vi "Main.vi"(11 "Module Admin":refnum<class "Delacor_lib_QMH_Cloneable Module Admin.lvclass">) -> ()   [LabVIEW 2020, in "TCP Client.lvlib"]
doc: "This template is based off of the Queued Message Handler design pattern and the Queued Message Handler project template that ships with LabVIEW.\n\nThe main difference is that the queue is private to this module and communication between modules is performed via Broadcast and Request events.\n\nRequest events are wrapped in public API methods and are handled in the Event Handling Loop (EHL) of this VI. Any module can register for Broadcast events sent by this module. The EHL generates messages based on user interface actions.\n\nThe Message Handling Loop (MHL) processes messages generated by the EHL, or by other messages. The messages are string values, so new messages can be added easily to the Message Cases case structure in the MHL. Each message cluster can also provide an optional value for Message Data, which is a variant that can be converted to whatever message-specific data is required.\n_____\nBased on DQMH Project Template 6.0.0.91."
uses:
  TCP Client.lvlib
  <vilib>/Delacor/Delacor QMH/Libraries/Cloneable Module Admin_class/Delacor_lib_QMH_Cloneable Module Admin.lvclass
  C:/Program Files (x86)/National Instruments/LabVIEW 2020/vi.lib/Delacor/Delacor QMH/Libraries/Module Admin_class/Delacor_lib_QMH_Module Admin.lvclass
  Module Data--cluster.ctl
  <vilib>/Delacor/Delacor QMH/Libraries/Message Queue_class/Delacor_lib_QMH_Message Queue.lvclass/Delacor_lib_QMH_Message Queue.ctl
  <vilib>/Delacor/Delacor QMH/Libraries/Cloneable Module Admin_class/Delacor_lib_QMH_Cloneable Module Admin.lvclass/Delacor_lib_QMH_Cloneable Module Admin.ctl
  Stop Argument--cluster.ctl
  <vilib>/Delacor/Delacor QMH/Libraries/Module Admin_class/Delacor_lib_QMH_Module Admin.lvclass/Delacor_lib_QMH_Module Admin.ctl
  <vilib>/Utility/miscctls.llb/LVPointTypeDef.ctl
  <vilib>/Delacor/Delacor QMH/Libraries/Message Queue_class/Delacor_lib_QMH_Enqueue Message (Single).vi
  <vilib>/Delacor/Delacor QMH/Libraries/Cloneable Module Admin_class/Delacor_lib_QMH_Get Module ID.vi
  <vilib>/Delacor/Delacor QMH/Libraries/Module Admin_class/Delacor_lib_QMH_Get External Launch.vi
  <vilib>/Utility/error.llb/Error Cluster From Error Code.vi
  <vilib>/ErrorRing/Error Ring.xnode
  <vilib>/Delacor/Delacor QMH/Libraries/Message Queue_class/Delacor_lib_QMH_Message Queue.lvclass
panel:
  out "Data":T1 {"Knob" scale=0.0..10.0; "Slide" scale=0.0..10.0}
  out "error out":errorcluster
  out "Status":string
  in  "Simulate EHL Error":bool
  in  "Simulate MHL Error":bool
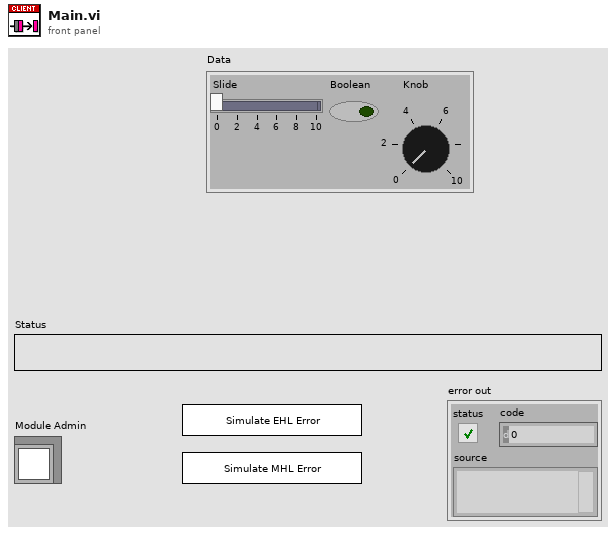
[diagram p1: front panel]
types:
  T1 = cluster{"Slide":dbl, "Boolean":bool, "Knob":dbl, "Selector":i32}
  T2 = typedef "TCP Client.lvlib/Request Events--cluster.ctl" = cluster{"Stop Module":refnum<user-event>, "Show Panel":refnum<user-event>, "Hide Panel":refnum<user-event>, "Show Diagram":refnum<user-event>, "Get Module Execution Status":refnum<user-event>, "Connect To TCP Server":refnum<user-event>, "Choose selector":refnum<user-event>}
  T3 = typedef "TCP Client.lvlib/Module Data--cluster.ctl" = cluster{"Status":string}
  T4 = enum32{"invalid lock state", "Not Locked", "Locked (No Password)", "Password-protected"}
  T5 = typedef "TCP Client.lvlib/Stop Argument--cluster.ctl" = cluster{"Module ID":i32, "Origin":string, "Exit via Stop Module Req?":bool, "Wait for Module to stop?":bool}
  T6 = typedef "LVPointTypeDef.ctl" = cluster{"Horizontal":i16, "Vertical":i16}
  T7 = enum32{"Invalid", "Standard", "Closed", "Hidden", "Minimized", "Maximized"}
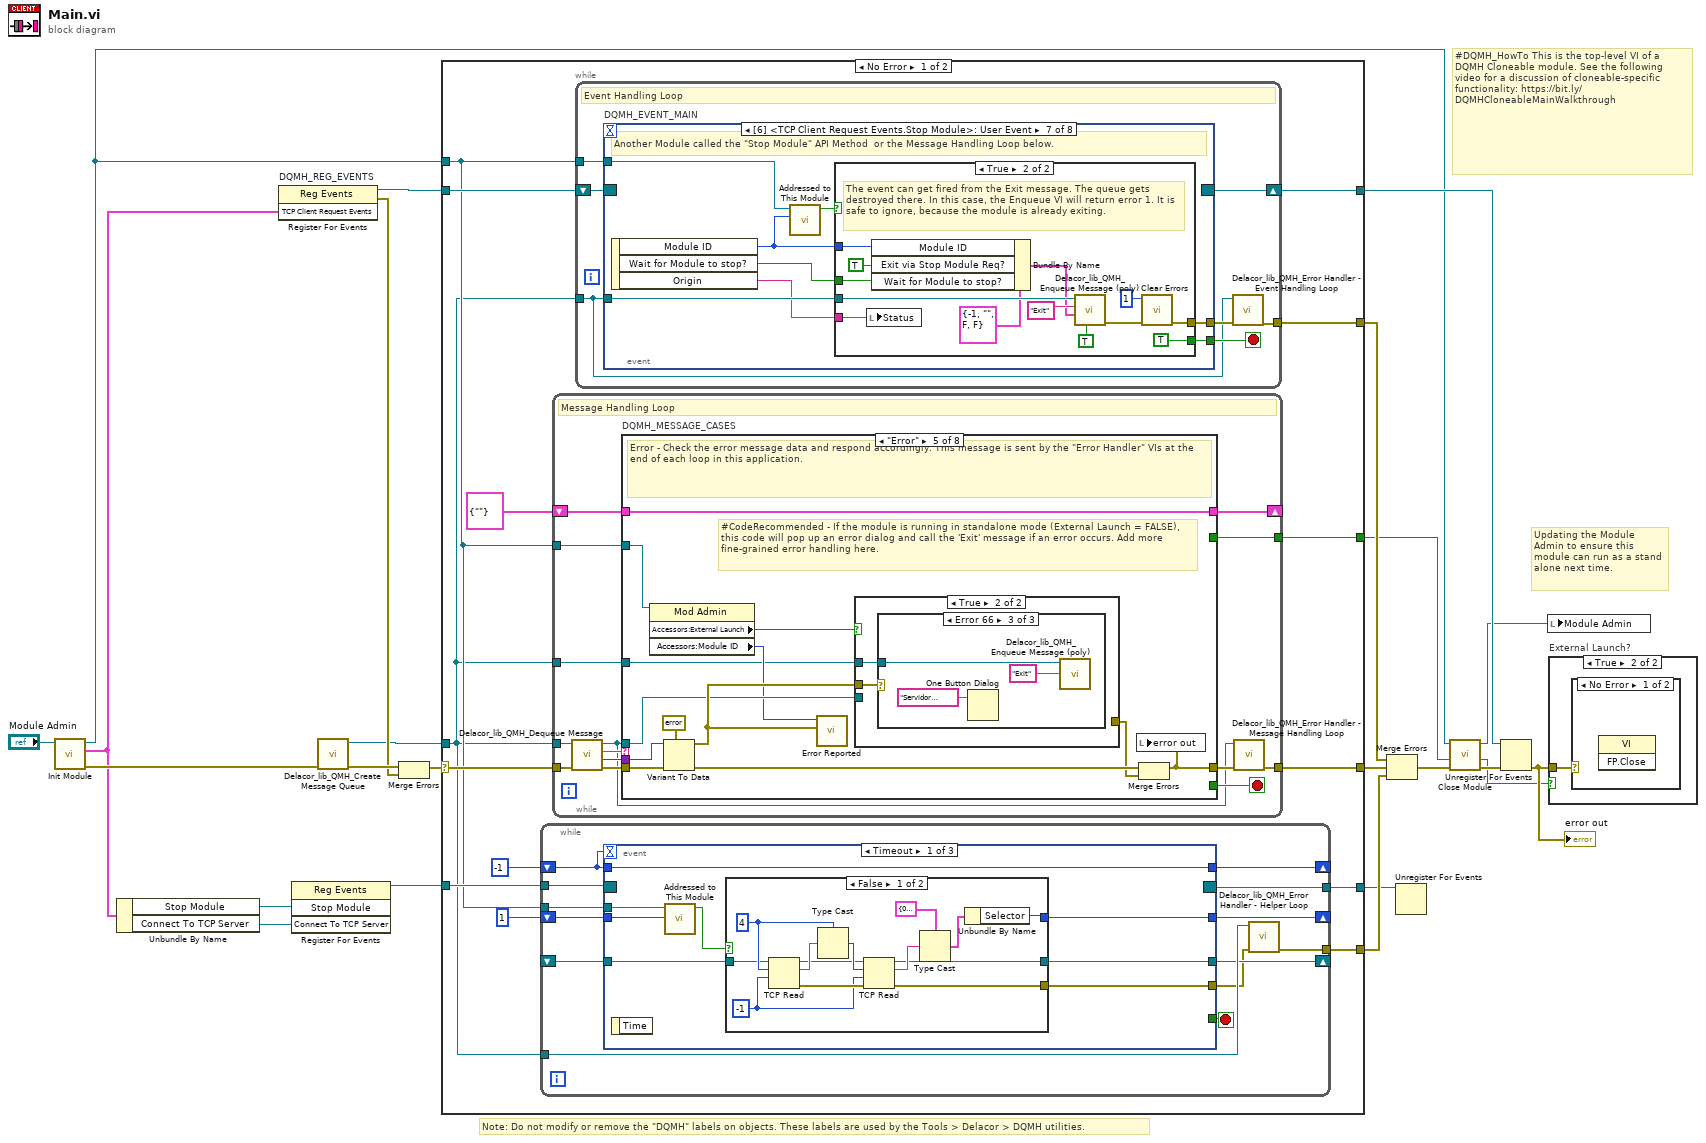
[diagram p0: block diagram]
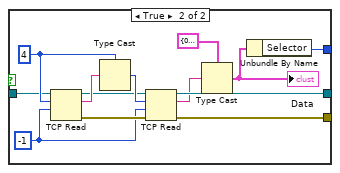
[diagram p2: hidden frame]
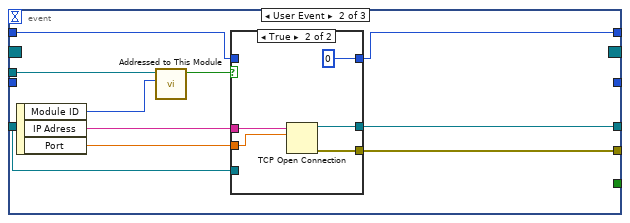
[diagram p3: hidden frame]
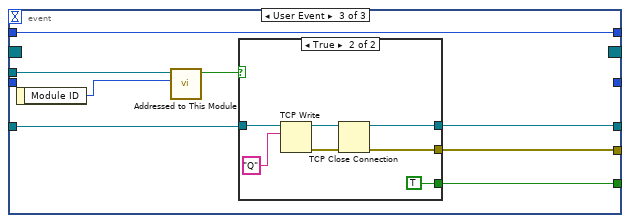
[diagram p5: hidden frame]
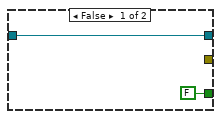
[diagram p6: hidden frame]
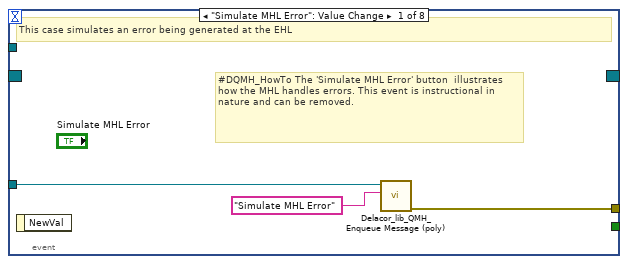
[diagram p7: hidden frame]
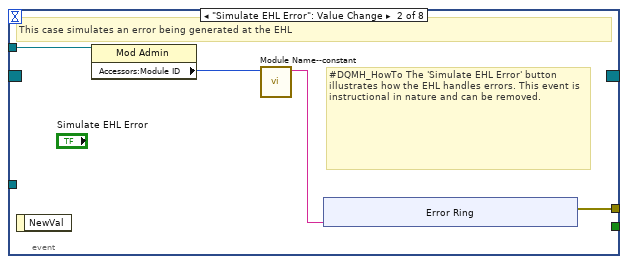
[diagram p8: hidden frame]
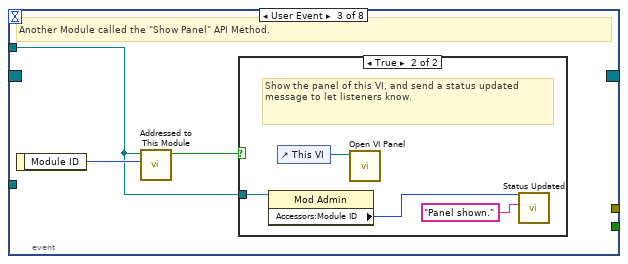
[diagram p9: hidden frame]
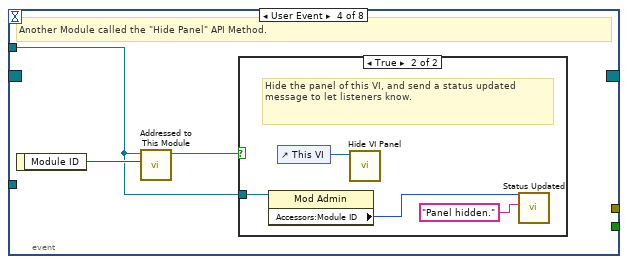
[diagram p11: hidden frame]
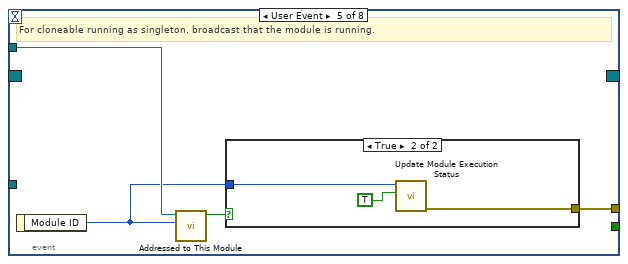
[diagram p13: hidden frame]
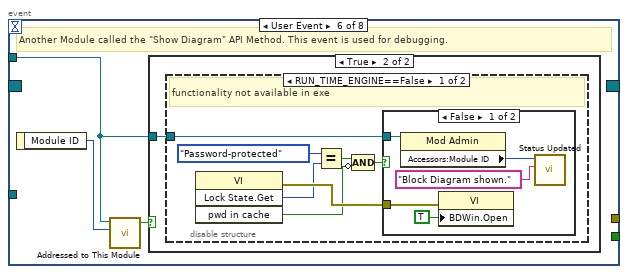
[diagram p15: hidden frame]
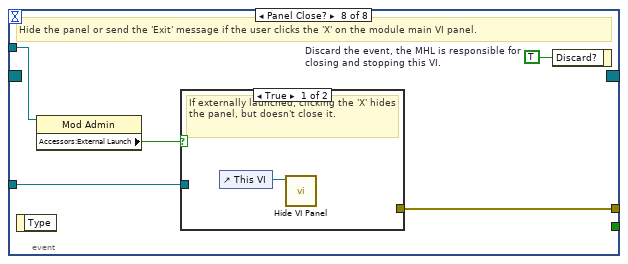
[diagram p20: hidden frame]
diagram:
  # "#DQMH_HowTo This is the top-level VI of a DQMH Cloneable module. See the following video for a discussion of cloneable-specific functionality: https://bit.ly/DQMHCloneableMainWalkthrough"
  # "Note: Do not modify or remove the \"DQMH\" labels on objects. These labels are used by the Tools > Delacor > DQMH utilities."
  # "Updating the Module Admin to ensure this module can run as a stand alone next time."
  n1 = call "Init Module.vi"("Cloneable Module Admin in"="Module Admin") -> ("error out"=w20:errorcluster, "TCP Client Request Events"=w6:T2, "Cloneable Module Admin out"=w10:refnum<class "Delacor_lib_QMH_Cloneable Module Admin.lvclass">)  [unwired: 8 in]
  n2 = Unbundle By Name(w6) -> ("Stop Module"=w5:refnum<user-event>, "Connect To TCP Server"=w3:refnum<user-event>)
  n3 = register-events "DQMH_REG_EVENTS"(w6) -> (reference out=w13:refnum<event-registration>, error out=w15:errorcluster)  [unwired: 2 in]
  n4 = register-events(w5, w3) -> (reference out=w4:refnum<event-registration>)  [unwired: 2 in, 1 out]
  n5 = call <vilib>:"Delacor_lib_QMH_Create Message Queue.vi"("error in"=w20) -> ("error out"=w17:errorcluster, "Message Queue"=w12:refnum<class "Delacor_lib_QMH_Message Queue.lvclass">)  [unwired: 9 in]
  n6 = Merge Errors(w17, w15) -> (w16:errorcluster)
  n7 = case shown="No Error" w16 {
    selector: w16 -> [w35 w321]
    tunnel: [w37 w320] -> w21
    tunnel: [w34 w328] -> w14
    tunnel: w13 -> [w32 w328]
    tunnel: w12 -> [w24 w319]
    tunnel: [w36 _] -> w22
    tunnel: w10 -> [w28 w324]
    tunnel: [w31 _] -> w8
    tunnel: w4 -> [w30 _]
    tunnel: [w29 _] -> w1
    tunnel: [w27 _] -> w2
    frame No Error {
      n8 = while {
        tunnel: w30 -> [w50]
        tunnel: [w49] -> w29
        tunnel: w24 -> [w47]
        tunnel: w28 -> [w46]
        tunnel: [w45] -> w27
        shift-right: [w44] -> _
        shift-left: _ -> [w42]
        shift-right: [w41] -> _
        shift-left: -1 -> [w40]
        shift-right: [w38] -> _
        shift-left: 1 ("Selector") -> [w39]
        stop <- w48 stop-if-true
        n9 = event shown="[0] Timeout" {
          selector: w50 -> [_ _ _]
          dyn-events: [_ _ _] -> w49
          timeout: w40 -> [_ _ _]
          tunnel: [_ _ w102] -> w48
          tunnel: w46 -> [w56 w87 w105]
          tunnel: [w52 w92 w107] -> w44
          tunnel: [w53 w91 w106] -> w43
          tunnel: w42 -> [w57 w90 w108]
          tunnel: [w58 w88 w109] -> w41
          tunnel: w40 -> [w58 w89 w109]
          tunnel: w39 -> [w54 _ _]
          tunnel: [w51 _ _] -> w38
          event Timeout {
            n10 = event-data() -> ()  [unwired: 1 in, 1 out]
            n11 = call "Addressed to This Module.vi"("Module ID from Argument"=w54, "Module Admin"=w56) -> ("Addressed to this instance?"=w55:bool)  [unwired: 8 in, 1 out]
            n12 = case shown="False" w55 {
              tunnel: w57 -> [w62 w78]
              tunnel: [w60 w77] -> w53
              tunnel: [w61 w76] -> w52
              tunnel: [w59 w72] -> w51
              frame False {
                w66 = -1
                w67 = 4
                n13 = TCP Read(connection ID=w62, bytes to read=w67, 9:w66) -> (connection ID out=w68:refnum<k5>, data out=w71:string, error out=w70:errorcluster)  [unwired: 1 in, 1 out]
                n14 = Type Cast(type=w67, x=w71) -> (*(type *) &x=w69:i32)
                n15 = TCP Read(connection ID=w68, bytes to read=w69, error in (no error)=w70, 9:w66) -> (connection ID out=w61:refnum<k5>, data out=w65:string, error out=w60:errorcluster)  [unwired: 1 out]
                n16 = Type Cast(type=T1 {"Slide"=0.0, "Boolean"=FALSE, "Knob"=0.0, "Selector"=0} ("Data"), x=w65) -> (*(type *) &x=w63:T1)
                n17 = Unbundle By Name(w63) -> ("Selector"=w59:i32)
              }
              frame True {
                w79 = -1
                w80 = 4
                n18 = TCP Read(connection ID=w78, bytes to read=w80, 9:w79) -> (connection ID out=w81:refnum<k5>, data out=w84:string, error out=w83:errorcluster)  [unwired: 1 in, 1 out]
                n19 = Type Cast(type=w80, x=w84) -> (*(type *) &x=w82:i32)
                n20 = TCP Read(connection ID=w81, bytes to read=w82, error in (no error)=w83, 9:w79) -> (connection ID out=w76:refnum<k5>, data out=w75:string, error out=w77:errorcluster)  [unwired: 1 out]
                n21 = Type Cast(type=T1 {"Slide"=0.0, "Boolean"=FALSE, "Knob"=0.0, "Selector"=0} ("Data"), x=w75) -> (*(type *) &x=w73:T1)
                "Data" <- w73
                n22 = Unbundle By Name(w73) -> ("Selector"=w72:i32)
              }
            }
          }
          event User Event {
            n23 = event-data() -> ("Module ID"=w85:i32, "IP Adress"=w94:string, "Port"=w93:dbl)  [unwired: 1 in]
            n24 = call "Addressed to This Module.vi"("Module ID from Argument"=w85, "Module Admin"=w87) -> ("Addressed to this instance?"=w86:bool)  [unwired: 8 in, 1 out]
            n25 = case shown="True" w86 {
              tunnel: w94 -> [_ w101]
              tunnel: w93 -> [_ w100]
              tunnel: [w96 w99] -> w92
              tunnel: [_ w98] -> w91
              tunnel: w90 -> [w96 _]
              tunnel: w89 -> [w95 _]
              tunnel: [w95 0] -> w88
              frame False {
              }
              frame True {
                n26 = TCP Open Connection(address=w101, remote port or service name=w100) -> (connection ID=w99:refnum<k5>, error out=w98:errorcluster)  [unwired: 1 in, 2 out]
              }
            }
          }
          event User Event {
            n27 = event-data() -> ("Module ID"=w104:i32)  [unwired: 1 in]
            n28 = call "Addressed to This Module.vi"("Module ID from Argument"=w104, "Module Admin"=w105) -> ("Addressed to this instance?"=w103:bool)  [unwired: 8 in, 1 out]
            n29 = case shown="True" w103 {
              tunnel: w108 -> [w111 w117]
              tunnel: [w111 w114] -> w107
              tunnel: [_ w113] -> w106
              tunnel: [FALSE TRUE] -> w102
              frame False {
              }
              frame True {
                n30 = TCP Write(connection ID=w117, data in="Q") -> (connection ID out=w116:refnum<k5>, error out=w115:errorcluster)  [unwired: 1 in, 2 out]
                n31 = TCP Close Connection(connection ID=w116, error in (no error)=w115) -> (connection ID out=w114:refnum<k5>, error out=w113:errorcluster)  [unwired: 1 out]
              }
            }
          }
        }
        n32 = call-dynamic "Delacor_lib_QMH_Error Handler - Helper Loop.vi"("error in"=w43, "Message Queue in"=w47) -> ("dup error in"=w45:errorcluster)  [unwired: 8 in, 1 out]
      }
      n33 = while {
        tunnel: w24 -> [w212]
        shift-right: [w216] -> _
        shift-left: T3 {"Status"=""} ("Data Cluster") -> [w217]
        tunnel: w35 -> [w220]
        tunnel: [w218] -> w37
        tunnel: w28 -> [w210]
        tunnel: [w209] -> w31
        tunnel: w24 -> [w208]
        stop <- w215 stop-if-true
        # "Message Handling Loop"
        n34 = call-dynamic "Delacor_lib_QMH_Dequeue Message.vi"("error in"=w220, "Message Queue in"=w212) -> ("error out"=w219:errorcluster, "Message Data"=w213:variant, "Message"=w214:string, "Message Queue out"=w211:refnum<class "Delacor_lib_QMH_Message Queue.lvclass">)  [unwired: 6 in]
        n35 = case "DQMH_MESSAGE_CASES" shown="\"Error\"" w214 {
          selector: w214 -> [_ _ _ _ _ _ _ w306]
          tunnel: w211 -> [_ _ _ _ w252 _ w296 _]
          tunnel: w219 -> [w240 w244 w247 w249 w261 w279 w302 w308]
          tunnel: [w238 w244 w246 w249 w257 w278 w299 w309] -> w221
          tunnel: w217 -> [w231 w243 w245 w248 w256 w276 w295 w307]
          tunnel: [w230 w243 w245 w248 w256 w276 w295 w307] -> w216
          tunnel: [_ _ _ _ _ _ w294 _] -> w215
          tunnel: w213 -> [_ _ _ _ w255 _ w292 _]
          tunnel: w210 -> [w225 _ _ _ w254 w274 w288 w304]
          tunnel: [_ _ _ _ _ _ w290 _] -> w209
          tunnel: w208 -> [_ _ _ _ w250 _ _ _]
          frame "Initialize" {
            w222 = "Initial Message" ("Initial Message")
            # "#CodeNeeded - Initialize the appearance of the front panel."
            # "#CodeNeeded - Initialize your state data here."
            # "Initialize - Any operation that needs to be done before the module can receive messages. Synchronize Caller Events.vi will inform Start Module.vi that the module has launched and is ready to receive messages. Module Did Init.vi will broadcast that the module initialized."
            n36 = call "Synchronize Caller Events.vi"("error in (no error)"=w240, "Module Admin"=w225) -> ("error out"=w239:errorcluster, "Module Admin out"=w224:refnum<class "Delacor_lib_QMH_Cloneable Module Admin.lvclass">)  [unwired: 8 in]
            n37 = property class="Mod Admin"(reference=w224) -> ("Accessors:Module ID"=w227:i32, "Accessors:External Launch"=w226:bool)  [unwired: 1 in, 2 out]
            n38 = call "Module Name--constant.vi"("Module ID"=w227) -> ("Module Name"=w235:string)  [unwired: 10 in]
            n39 = property class="VI"("Front Panel.Title"=w235) -> (reference out=w237:refnum<vi>, error out=w242:errorcluster)  [unwired: 2 in]
            n40 = Select(t=T7."Hidden" ("State"), s=w226, f=T7."Standard" ("State")) -> (s? t:f=w232:T7)
            n41 = invoke class="VI" method="FP.Open"(reference=w237, error in=w242, "State"=w232) -> (reference out=w236:refnum<vi>, error out=w241:errorcluster)  [unwired: 2 in, 3 out]
            n42 = call "Module Name--constant.vi"("Module ID"=w227) -> ("Module Name"=w228:string)  [unwired: 10 in]
            n43 = Bundle By Name(cluster=w231, "Status"=w222) -> (w230:T3)
            n44 = invoke class="VI" method="FP.Center"(reference=w236, error in=w241) -> ()  [unwired: 1 in, 3 out]
            n45 = property on="Pane" class="Pane"("Origin"=T6 {"Horizontal"=0, "Vertical"=0}) -> ()  [unwired: 2 in, 2 out]
            n46 = call "Module Did Init.vi"("error in (no error)"=w239, "Initialized?"=TRUE, "Origin"=w228, "Module ID"=w227) -> ("error out"=w238:errorcluster)  [unwired: 7 in]
            "Status" <- w222
          }
          frame "---Module Specific---" {
            # "Separator -- The following cases handle messages specific to this Module."
          }
          frame "---Copy This Frame---" {
            # "Duplicate this frame when creating new messages.  Change this comment in the duplicated frame to describe this message."
            n47 = Merge Errors(w247) -> (w246:errorcluster)
          }
          frame "---Exit and Error Handling---" {
            # "Separator - the following cases handle errors and exit messages."
          }
          frame "Error" {
            # "#CodeRecommended - If the module is running in standalone mode (External Launch = FALSE), this code will pop up an error dialog and call the 'Exit' message if an error occurs. Add more fine-grained error handling here."
            # "Error - Check the error message data and respond accordingly. This message is sent by the \"Error Handler\" VIs at the end of each loop in this application."
            n48 = property class="Mod Admin"(reference=w254) -> ("Accessors:External Launch"=w253:bool, "Accessors:Module ID"=w251:i32)  [unwired: 1 in, 2 out]
            n49 = Variant To Data(error in=w261, type=errorcluster {"status"=FALSE, "code"=0, "source"=""} ("error constant"), Variant=w255) -> (data=w262:errorcluster, error out=w259:errorcluster)
            n50 = call "Error Reported.vi"("Error"=w262, "Module ID"=w251) -> ()  [unwired: 9 in, 1 out]
            n51 = case shown="True" w253 {
              tunnel: [w267 _] -> w258
              tunnel: w252 -> [w265 _]
              tunnel: w262 -> [w266 w269]
              tunnel: w250 -> [_ w268]
              frame False {
                # "If the module is running standalone, then pop up an error dialog and call the \"Exit\" message."
                n52 = call <vilib>:"Simple Error Handler.vi"("error in (no error)"=w266) -> ()  [unwired: 4 in, 5 out]
                n53 = call-poly <vilib>:"Delacor_lib_QMH_Enqueue Message (poly).vi"("Priority Message? (F)"=TRUE, "Message"="Exit", "Message Queue in"=w265) -> ("error out"=w267:errorcluster)  [unwired: 7 in, 1 out]
              }
              frame True {
                n54 = case shown="Error 66" w269 {
                  tunnel: w268 -> [_ _ w270]
                  frame No Error {
                  }
                  frame Default {
                  }
                  frame Error {
                    n55 = One Button Dialog(message="Servidor desconectado") -> ()  [unwired: 1 in, 1 out]
                    n56 = call-poly <vilib>:"Delacor_lib_QMH_Enqueue Message (poly).vi"("Message"="Exit", "Message Queue in"=w270) -> ()  [unwired: 8 in, 2 out]
                  }
                }
              }
            }
            n57 = Merge Errors(w259, w258) -> (w257:errorcluster)
            n58 = local write "error out"(w257) -> ()
          }
          frame "Simulate MHL Error" {
            # "#DQMH_HowTo The 'Simulate MHL Error' button  illustrates how the MHL handles errors. This event is instructional in nature and can be removed."
            # "Simulate an error occurring at the MHL"
            n59 = property class="Mod Admin"(reference=w274) -> ("Accessors:Module ID"=w275:i32)  [unwired: 1 in, 2 out]
            n60 = call "Module Name--constant.vi"("Module ID"=w275) -> ("Module Name"=w273:string)  [unwired: 10 in]
            n61 = xnode "Error Ring"("parameter 0"=w273) -> ("error out"=w277:errorcluster)
            n62 = Merge Errors(w279, w277) -> (w278:errorcluster)
          }
          frame "Exit" {
            w293 = 91  # 91: not all Exit messages will have an argument
            w294 = TRUE  # Stop the VI
            # "Release the message queue reference"
            # "#CodeNeeded - Add any required cleanup code here."
            # "Exit - Exit the application."
            n63 = Variant To Data(error in=w302, type=T5 {"Module ID"=-1, "Origin"="", "Exit via Stop Module Req?"=FALSE, "Wait for Module to stop?"=FALSE} ("Stop Argument"), Variant=w292) -> (data=w289:T5, error out=w297:errorcluster)
            n64 = call <vilib>:"Clear Errors.vi"("error in (no error)"=w297, "specific error code to clear (0: all)"=w293) -> ("error out"=w301:errorcluster)  [unwired: 4 in, 1 out]
            n65 = control-ref of="This VI"() -> (w287:refnum<vi>)
            n66 = call-dynamic "Delacor_lib_QMH_Release Message Queue.vi"("error in"=w301, "Message Queue"=w296) -> ("error out"=w300:errorcluster)  [unwired: 9 in]
            n67 = call "Handle Exit.vi"("Stop Argument"=w289, "Module Admin in"=w288, "VI reference"=w287) -> ("error out"=w298:errorcluster, "Wait for Stop?"=w290:bool)  [unwired: 7 in]
            n68 = Merge Errors(w300, w298) -> (w299:errorcluster)
          }
          frame Default {
            # "'Default' case only runs if there is a message that isn't defined in any of the other cases.  Output a programming error."
            n69 = property class="Mod Admin"(reference=w304) -> ("Accessors:Module ID"=w303:i32)  [unwired: 1 in, 2 out]
            n70 = call "Module Name--constant.vi"("Module ID"=w303) -> ("Module Name"=w305:string)  [unwired: 10 in]
            n71 = xnode "Error Ring"("parameter 0"=w306, "parameter 1"=w305) -> ("error out"=w310:errorcluster)
            n72 = Merge Errors(w308, w310) -> (w309:errorcluster)
          }
        }
        n73 = call-dynamic "Delacor_lib_QMH_Error Handler - Message Handling Loop.vi"("error in"=w221, "Message Queue in"=w211) -> ("dup error in"=w218:errorcluster)  [unwired: 8 in, 1 out]
      }
      n74 = while {
        tunnel: w24 -> [w119]
        shift-right: [w122] -> w34
        shift-left: w32 -> [w123]
        tunnel: [w124] -> w36
        tunnel: w28 -> [w120]
        stop <- w121 stop-if-true
        # "Event Handling Loop"
        n75 = event "DQMH_EVENT_MAIN" shown="[6] <TCP Client Request Events.Stop Module>: User Event" {
          selector: w123 -> [_ _ _ _ _ _ _ _]
          dyn-events: [_ _ _ _ _ _ _ _] -> w122
          timeout: _ -> [_ _ _ _ _ _ _ _]
          tunnel: [_ _ _ _ _ _ w180 _] -> w121
          tunnel: w119 -> [w127 _ _ _ _ _ w183 w199]
          tunnel: [w128 w132 _ _ w157 _ w184 w202] -> w125
          tunnel: w120 -> [_ w131 w140 w147 w155 w161 w182 w200]
          event "Simulate MHL Error": Value Change {
            # "#DQMH_HowTo The 'Simulate MHL Error' button  illustrates how the MHL handles errors. This event is instructional in nature and can be removed."
            # "This case simulates an error being generated at the EHL"
            n76 = event-data() -> ()  [unwired: 1 in, 1 out]
            n77 = call-poly <vilib>:"Delacor_lib_QMH_Enqueue Message (poly).vi"("Message"="Simulate MHL Error", "Message Queue in"=w127) -> ("error out"=w128:errorcluster)  [unwired: 8 in, 1 out]
          }
          event "Simulate EHL Error": Value Change {
            # "#DQMH_HowTo The 'Simulate EHL Error' button  illustrates how the EHL handles errors. This event is instructional in nature and can be removed."
            # "This case simulates an error being generated at the EHL"
            n78 = event-data() -> ()  [unwired: 1 in, 1 out]
            n79 = property class="Mod Admin"(reference=w131) -> ("Accessors:Module ID"=w130:i32)  [unwired: 1 in, 2 out]
            n80 = call "Module Name--constant.vi"("Module ID"=w130) -> ("Module Name"=w129:string)  [unwired: 10 in]
            n81 = xnode "Error Ring"("parameter 0"=w129) -> ("error out"=w132:errorcluster)
          }
          event User Event {
            # "Another Module called the \"Show Panel\" API Method."
            n82 = event-data() -> ("Module ID"=w141:i32)  [unwired: 1 in]
            n83 = call "Addressed to This Module.vi"("Module ID from Argument"=w141, "Module Admin"=w140) -> ("Addressed to this instance?"=w142:bool)  [unwired: 8 in, 1 out]
            n84 = case shown="True" w142 {
              tunnel: w140 -> [_ w144]
              frame False {
              }
              frame True {
                # "Show the panel of this VI, and send a status updated message to let listeners know."
                n85 = property class="Mod Admin"(reference=w144) -> ("Accessors:Module ID"=w143:i32)  [unwired: 1 in, 2 out]
                n86 = control-ref of="This VI"() -> (w146:refnum<vi>)
                n87 = call "Open VI Panel.vi"("VI"=w146) -> ()  [unwired: 10 in, 1 out]
                n88 = call "Status Updated.vi"("Status"="Panel shown." ("format string"), "Module ID"=w143) -> ()  [unwired: 9 in, 1 out]
              }
            }
          }
          event User Event {
            # "Another Module called the \"Hide Panel\" API Method."
            n89 = event-data() -> ("Module ID"=w148:i32)  [unwired: 1 in]
            n90 = call "Addressed to This Module.vi"("Module ID from Argument"=w148, "Module Admin"=w147) -> ("Addressed to this instance?"=w149:bool)  [unwired: 8 in, 1 out]
            n91 = case shown="True" w149 {
              tunnel: w147 -> [_ w151]
              frame False {
              }
              frame True {
                # "Hide the panel of this VI, and send a status updated message to let listeners know."
                n92 = property class="Mod Admin"(reference=w151) -> ("Accessors:Module ID"=w150:i32)  [unwired: 1 in, 2 out]
                n93 = control-ref of="This VI"() -> (w153:refnum<vi>)
                n94 = call "Hide VI Panel.vi"("VI"=w153) -> ()  [unwired: 10 in, 1 out]
                n95 = call "Status Updated.vi"("Status"="Panel hidden." ("format string"), "Module ID"=w150) -> ()  [unwired: 9 in, 1 out]
              }
            }
          }
          event User Event {
            # "For cloneable running as singleton, broadcast that the module is running."
            n96 = event-data() -> ("Module ID"=w154:i32)  [unwired: 1 in]
            n97 = call "Addressed to This Module.vi"("Module ID from Argument"=w154, "Module Admin"=w155) -> ("Addressed to this instance?"=w156:bool)  [unwired: 8 in, 1 out]
            n98 = case shown="True" w156 {
              tunnel: [_ w160] -> w157
              tunnel: w154 -> [_ w159]
              frame False {
              }
              frame True {
                n99 = call "Update Module Execution Status.vi"("Running?"=TRUE, "Module ID"=w159) -> ("error out"=w160:errorcluster)  [unwired: 9 in]
              }
            }
          }
          event User Event {
            # "Another Module called the \"Show Diagram\" API Method. This event is used for debugging."
            n100 = event-data() -> ("Module ID"=w162:i32)  [unwired: 1 in]
            n101 = call "Addressed to This Module.vi"("Module ID from Argument"=w162, "Module Admin"=w161) -> ("Addressed to this instance?"=w163:bool)  [unwired: 8 in, 1 out]
            n102 = case shown="True" w163 {
              tunnel: w161 -> [_ w164]
              frame False {
              }
              frame True {
                n103 = disable-structure shown="RUN_TIME_ENGINE==False" {
                  disable-tunnel: w164 -> [w165 _]
                  frame condition #0 (active) {
                    # "functionality not available in exe"
                    n104 = invoke class="VI" method="Lock State.Get"() -> (error out=w171:errorcluster, "Get Lock State"=w170:T4, "pwd in cache"=w167:bool)  [unwired: 4 in, 1 out]
                    n105 = Equal?(x=T4."Password-protected", y=w170) -> (x = y?=w168:bool)
                    n106 = Compound Arithmetic op=AND(w168, invert w167) -> (w166:bool)
                    n107 = case shown="False" w166 {
                      tunnel: w171 -> [w176 _]
                      tunnel: w165 -> [w173 _]
                      frame False {
                        n108 = property class="Mod Admin"(reference=w173) -> ("Accessors:Module ID"=w172:i32)  [unwired: 1 in, 2 out]
                        n109 = property class="VI"(error in=w176, "BDWin.Open"=TRUE ("Block Diagram Window:Open")) -> ()  [unwired: 1 in, 2 out]
                        n110 = call "Status Updated.vi"("Status"="Block Diagram shown." ("format string"), "Module ID"=w172) -> ()  [unwired: 9 in, 1 out]
                      }
                      frame True {
                        # "Password-protected VI, and the password is not in the cache. Do not show the diagram."
                      }
                    }
                  }
                  frame condition #1 {
                  }
                }
              }
            }
          }
          event User Event {
            # "Another Module called the \"Stop Module\" API Method  or the Message Handling Loop below."
            n111 = event-data() -> ("Module ID"=w178:i32, "Wait for Module to stop?"=w179:bool, "Origin"=w177:string)  [unwired: 1 in]
            n112 = call "Addressed to This Module.vi"("Module ID from Argument"=w178, "Module Admin"=w182) -> ("Addressed to this instance?"=w181:bool)  [unwired: 8 in, 1 out]
            n113 = case shown="True" w181 {
              tunnel: [_ w196] -> w184
              tunnel: w183 -> [_ w192]
              tunnel: [_ TRUE] -> w180
              tunnel: w179 -> [_ w187]
              tunnel: w178 -> [_ w189]
              tunnel: w177 -> [_ w185]
              frame False {
              }
              frame True {
                # "The event can get fired from the Exit message. The queue gets destroyed there. In this case, the Enqueue VI will return error 1. It is safe to ignore, because the module is already exiting."
                n114 = local write "Status"(w185) -> ()
                n115 = Bundle By Name(cluster=T5 {"Module ID"=-1, "Origin"="", "Exit via Stop Module Req?"=FALSE, "Wait for Module to stop?"=FALSE} ("Stop Argument"), "Module ID"=w189, "Exit via Stop Module Req?"=TRUE, "Wait for Module to stop?"=w187) -> (w186:T5)
                n116 = call-poly <vilib>:"Delacor_lib_QMH_Enqueue Message (poly).vi"("Priority Message? (F)"=TRUE, "Message Data"=w186, "Message"="Exit", "Message Queue in"=w192) -> ("error out"=w197:errorcluster)  [unwired: 6 in, 1 out]
                n117 = call <vilib>:"Clear Errors.vi"("error in (no error)"=w197, "specific error code to clear (0: all)"=1) -> ("error out"=w196:errorcluster)  [unwired: 4 in, 1 out]
              }
            }
          }
          event Panel Close? {
            w201 = TRUE  # Discard the event, the MHL is responsible for closing and stopping this VI.
            # "Hide the panel or send the 'Exit' message if the user clicks the 'X' on the module main VI panel."
            n118 = event-data() -> ()  [unwired: 1 in, 1 out]
            n119 = property class="Mod Admin"(reference=w200) -> ("Accessors:External Launch"=w198:bool)  [unwired: 1 in, 2 out]
            n120 = case shown="True" w198 {
              tunnel: w199 -> [_ w206]
              tunnel: [_ w207] -> w202
              frame True {
                # "If externally launched, clicking the 'X' hides the panel, but doesn't close it."
                n121 = control-ref of="This VI"() -> (w203:refnum<vi>)
                n122 = call "Hide VI Panel.vi"("VI"=w203) -> ()  [unwired: 10 in, 1 out]
              }
              frame False {
                # "If run as a stand-alone VI, clicking the panel 'X' stops the VI."
                n123 = call-poly <vilib>:"Delacor_lib_QMH_Enqueue Message (poly).vi"("Priority Message? (F)"=TRUE, "Message"="Exit", "Message Queue in"=w206) -> ("error out"=w207:errorcluster)  [unwired: 7 in, 1 out]
              }
            }
            n124 = event-data("Discard?"=w201) -> ()  [unwired: 1 in, 1 out]
          }
        }
        n125 = call-dynamic "Delacor_lib_QMH_Error Handler - Event Handling Loop.vi"("error in"=w125, "Message Queue in"=w119) -> ("dup error in"=w124:errorcluster)  [unwired: 8 in, 1 out]
      }
    }
    frame Error {
      n126 = call "Synchronize Caller Events.vi"("Module Admin"=w324) -> ("Module Admin out"=w323:refnum<class "Delacor_lib_QMH_Cloneable Module Admin.lvclass">)  [unwired: 9 in, 1 out]
      n127 = property class="Mod Admin"(reference=w323) -> ("Accessors:Module ID"=w322:i32)  [unwired: 1 in, 2 out]
      n128 = call-dynamic "Delacor_lib_QMH_Release Message Queue.vi"("error in"=w321, "Message Queue"=w319) -> ("error out"=w320:errorcluster)  [unwired: 9 in]
      n129 = call "Module Name--constant.vi"("Module ID"=w322) -> ("Module Name"=w327:string)  [unwired: 10 in]
      n130 = Format Into String(format string="An error occurred during initialization. %s is no longer running.", w327) -> (resulting string=w325:string)  [unwired: 2 in, 1 out]
      n131 = call "Error Reported.vi"("Additional Information"=w325, "Error"=w320, "Module ID"=w322) -> ()  [unwired: 8 in, 1 out]
    }
  }
  n132 = Merge Errors(w22, w21, w2) -> (w23:errorcluster)
  n133 = Unregister For Events(event registration refnum=w1) -> ()  [unwired: 1 in, 1 out]
  n134 = call "Close Module.vi"("error in"=w23, "Wait for stop?"=w8, "Module Admin in"=w10) -> ("error out"=w19:errorcluster, "External Launch"=w7:bool, "Module Admin out"=w9:refnum<class "Delacor_lib_QMH_Cloneable Module Admin.lvclass">)  [unwired: 6 in]
  n135 = Unregister For Events(event registration refnum=w14, error in=w19) -> (error out=w18:errorcluster)
  "error out" <- w18
  n136 = local write "Module Admin"(w9) -> ()
  n137 = case "External Launch?" shown="True" w7 {
    tunnel: w18 -> [_ w329]
    frame False {
    }
    frame True {
      n138 = case shown="No Error" w329 {
        frame No Error {
          n139 = invoke class="VI" method="FP.Close"() -> ()  [unwired: 3 in, 3 out]
        }
        frame Error {
          n140 = invoke class="VI" method="FP.Open"("Activate"=TRUE ("Activate?")) -> ()  [unwired: 4 in, 5 out]
        }
      }
    }
  }
